vi "Merge.vi"(10 "Array 2":cluster{"Key":string, "Value":variant}[](array[cluster]), 11 "Array 1":cluster{"Key":string, "Value":variant}[](array[cluster])) -> (3 "Array":cluster{"Key":string, "Value":variant}[](array[cluster]))   [LabVIEW 2019, in "UI Common.lvlib"]
uses:
  UI Common.lvlib
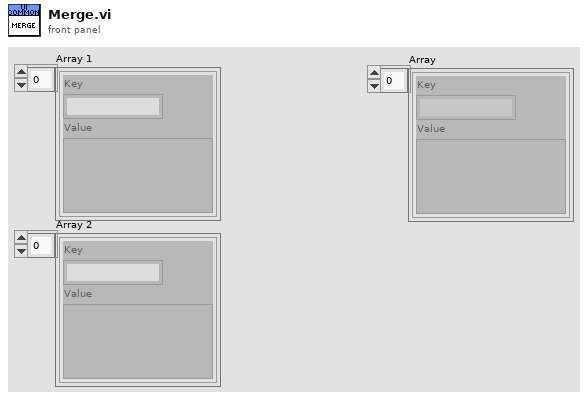
[diagram p1: front panel]
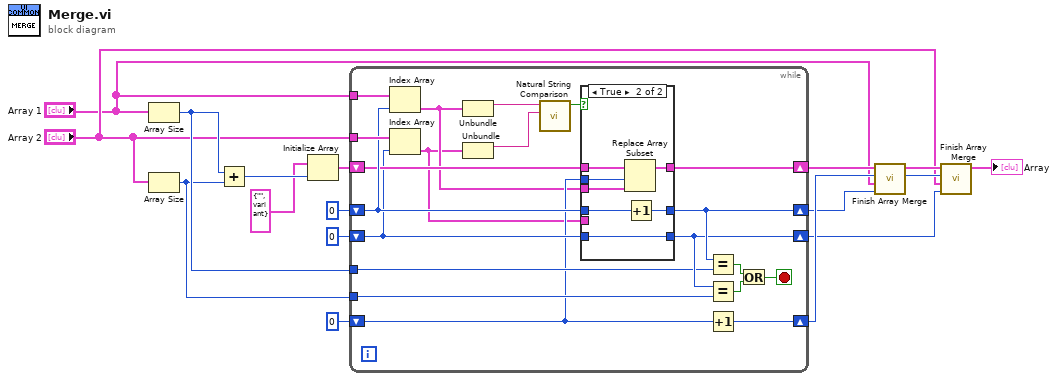
[diagram p0: block diagram]
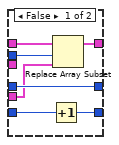
[diagram p2: hidden frame]
diagram:
  n1 = Array Size(array="Array 1") -> (size(s)=w12:i32)
  n2 = Array Size(array="Array 2") -> (size(s)=w11:i32)
  n3 = Add(x=w12, y=w11) -> (x+y=w17:i32)
  n4 = Initialize Array(cluster{"Key":string, "Value":variant} {"Key"="", "Value"=variant} ("Cluster"), w17) -> (w16:cluster{"Key":string, "Value":variant}[])
  n5 = while {
    shift-right: [w33] -> w13
    shift-left: w16 -> [w34]
    tunnel: w12 -> [w28]
    tunnel: w11 -> [w27]
    shift-right: [w31] -> w8
    shift-left: 0 -> [w35]
    shift-right: [w30] -> w5
    shift-left: 0 -> [w32]
    tunnel: "Array 1" -> [w37]
    tunnel: "Array 2" -> [w36]
    shift-right: [w23] -> w9
    shift-left: 0 -> [w24]
    stop <- w29 stop-if-true
    n6 = Index Array(array=w37, index=w35) -> (element=w19:cluster{"Key":string, "Value":variant})
    n7 = Index Array(array=w36, index=w32) -> (element=w18:cluster{"Key":string, "Value":variant})
    n8 = Unbundle(w19) -> ("Key"=w20:string)  [unwired: 1 out]
    n9 = Unbundle(w18) -> ("Key"=w21:string)  [unwired: 1 out]
    n10 = call "Natural String Comparison.vi"("String 2"=w21, "String 1"=w20) -> ("String 1 <= String 2"=w22:bool)  [unwired: 9 in]
    n11 = case shown="True" w22 {
      tunnel: w35 -> [w40 w49]
      tunnel: w34 -> [w44 w51]
      tunnel: [w43 w50] -> w33
      tunnel: w32 -> [w42 w47]
      tunnel: [w40 w48] -> w31
      tunnel: [w41 w47] -> w30
      tunnel: w19 -> [_ w46]
      tunnel: w18 -> [w39 _]
      tunnel: w24 -> [w38 w45]
      frame False {
        n12 = Increment(x=w42) -> (x+1=w41:i32)
        n13 = Replace Array Subset(array=w44, new element=w39, index=w38) -> (w43:cluster{"Key":string, "Value":variant}[])
      }
      frame True {
        n14 = Replace Array Subset(array=w51, new element=w46, index=w45) -> (w50:cluster{"Key":string, "Value":variant}[])
        n15 = Increment(x=w49) -> (x+1=w48:i32)
      }
    }
    n16 = Equal?(x=w31, y=w28) -> (x = y?=w26:bool)
    n17 = Equal?(x=w30, y=w27) -> (x = y?=w25:bool)
    n18 = Increment(x=w24) -> (x+1=w23:i32)
    n19 = Or(x=w26, y=w25) -> (x .or. y?=w29:bool)
  }
  n20 = call "Finish Array Merge.vi"("Array to Finish Index"=w8, "Array to Finish"="Array 1", "Result Index in"=w9, "Result Array in"=w13) -> ("Result Index out"=w6:i32, "Result Array out"=w7:cluster{"Key":string, "Value":variant}[])  [unwired: 6 in]
  n21 = call "Finish Array Merge.vi"("Array to Finish Index"=w5, "Array to Finish"="Array 2", "Result Index in"=w6, "Result Array in"=w7) -> ("Result Array out"=→"Array":cluster{"Key":string, "Value":variant}[])  [unwired: 6 in, 1 out]
